vi "Camera Global.vi"() -> ()   [LabVIEW 2013]
panel:
  in  "I (Front Camera)":dbl
  in  "D (Front Camera)":dbl
  in  "P (Front Camera)":dbl
  in  "Front Camera":T1
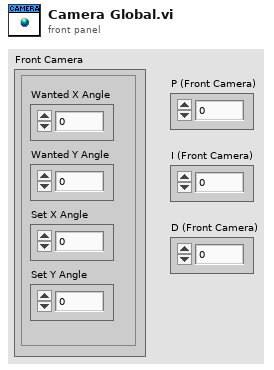
[diagram p1: front panel]
types:
  T1 = cluster{"Wanted X Angle":dbl, "Wanted Y Angle ":dbl, "Set X Angle":dbl, "Set Y Angle ":dbl}
diagram:
